vi "Intake Close Immediate.vi"(7 "Description":string, 8 "Command Info In":T1) -> (0 "Command Info Out":T1)   [LabVIEW 2017]
doc: "This template is useful for immediate subsystem actions that do not need deadband filtering\n\nBe sure to right-click and select New from Template and save with a new command name."
uses:
  <vilib>/Rock Robotics/WPI/Framework/Command Status Info.ctl
  <vilib>/Rock Robotics/WPI/Framework/Completion Status.ctl
  <vilib>/Rock Robotics/WPI/Framework/Completion Notifier.ctl
  Implementation/Intake Wheels Setpoints.ctl
  Implementation/Intake Wheels Operations.ctl
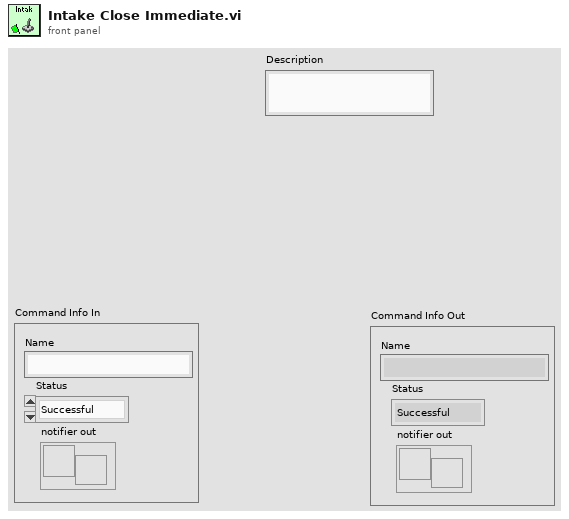
[diagram p1: front panel]
types:
  T1 = typedef "Command Status Info.ctl" = cluster{"Name":string, "Status":T2, "notifier out":T3}
  T2 = typedef "Completion Status.ctl" = enum16{"Successful", "Aborted", "Incomplete"}
  T3 = typedef "Completion Notifier.ctl" = refnum<notifier>
  T4 = typedef "Intake Wheels Setpoints.ctl" = cluster{"Operation":T5, "Left Wheel":dbl, "Duration":dbl, "Right Wheel":dbl}
  T5 = typedef "Intake Wheels Operations.ctl" = enum16{"Reserve", "Read Current", "Immediate", "Intake Open", "Intake Close", "Wheels On"}
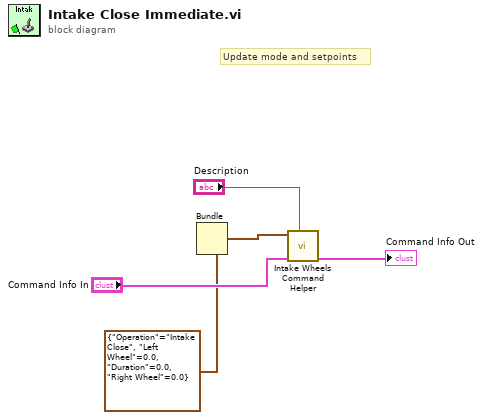
[diagram p0: block diagram]
diagram:
  # "Update mode and setpoints"
  n1 = Bundle(cluster=T4 {"Operation"=enum."Intake Close", "Left Wheel"=0.0, "Duration"=0.0, "Right Wheel"=0.0} ("SubSystem Data")) -> (w1:T4)  [unwired: 4 in]
  n2 = call "Intake Wheels Command Helper.vi"("Description"="Description", "Command Info In"="Command Info In", "SubSystem Data"=w1) -> ("Command Info Out"=→"Command Info Out":T1)  [unwired: 6 in, 2 out]
